vi "stateChange.vi"(8 "error in (no error)":errorcluster, 11 "StaticOutputEditor in":refnum<class "StaticOutputEditor.lvclass">) -> (0 "error out":errorcluster, 3 "StaticOutputEditor out":refnum<class "StaticOutputEditor.lvclass">)   [LabVIEW 2011, in "Views.lvlib" / "ScriptEditor.lvlib" / "StaticOutputEditor.lvclass"]
uses:
  StaticOutputEditor.lvclass
  StaticOutputEditor.lvclass/StaticOutputEditor.ctl
  Tools/DatabaseHelpers/Database Objects/ChannelArray/ChannelArray.lvclass
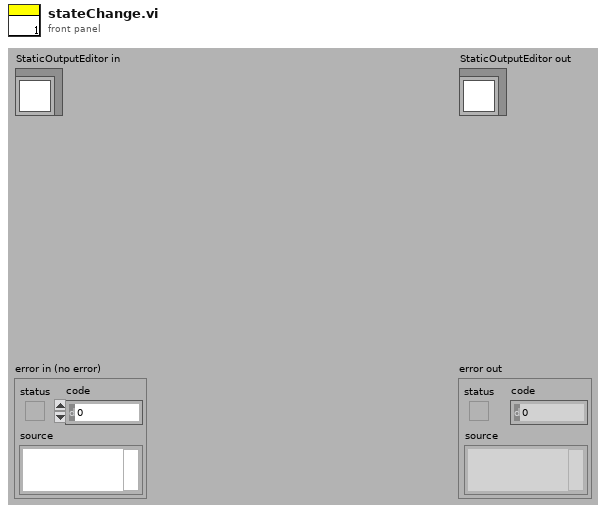
[diagram p1: front panel]
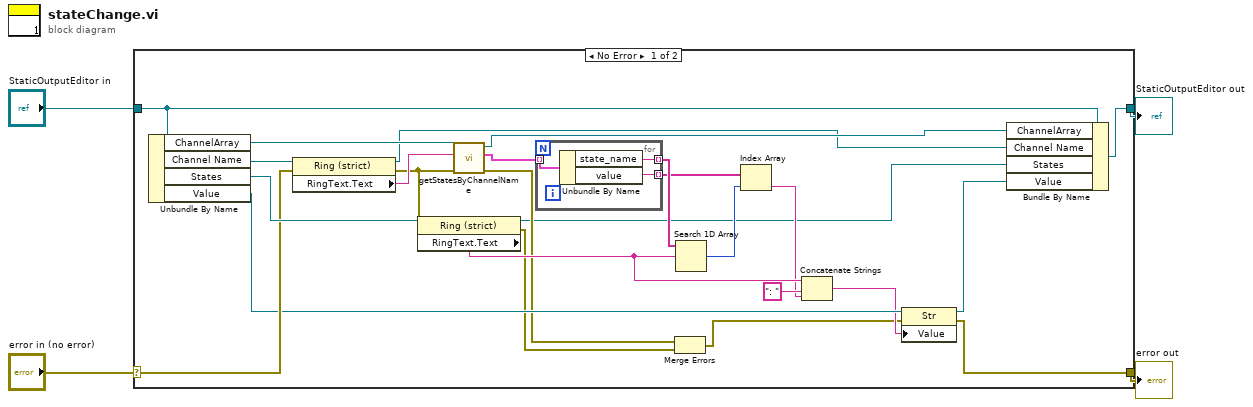
[diagram p0: block diagram]
diagram:
  n1 = case shown="No Error" "error in (no error)" {
    selector: "error in (no error)" -> [w24 w34]
    tunnel: [w11 w34] -> w3
    tunnel: [w5 w33] -> w1
    tunnel: "StaticOutputEditor in" -> [w6 w33]
    frame No Error {
      n2 = Unbundle By Name(w6) -> ("ChannelArray"=w28:refnum<class "ChannelArray.lvclass">, "Channel Name"=w27:refnum<vi>, "States"=w29:refnum<vi>, "Value"=w16:refnum<vi>)
      n3 = property class="Ring (strict)"(reference=w27, error in=w24) -> (reference out=w9:refnum<vi>, error out=w25:errorcluster, "RingText.Text"=w26:string)
      n4 = property class="Ring (strict)"(reference=w29, error in=w25) -> (reference out=w8:refnum<vi>, error out=w13:errorcluster, "RingText.Text"=w19:string)
      n5 = call "getStatesByChannelName.vi"("error in (no error)"=w25, "channel_name"=w26, "ChannelArray in"=w28) -> ("error out"=w14:errorcluster, "states"=w23:cluster{"state_name":string, "value":string}[], "ChannelArray out"=w10:refnum<class "ChannelArray.lvclass">)  [unwired: 6 in]
      n6 = for {
        tunnel: w23 -> [w32] mode=indexing
        tunnel: [w31] -> w22 mode=indexing
        tunnel: [w30] -> w21 mode=indexing
        n7 = Unbundle By Name(w32) -> ("state_name"=w31:string, "value"=w30:string)
      }
      n8 = Merge Errors(w14, w13) -> (w12:errorcluster)
      n9 = Search 1D Array(1D array=w22, element=w19) -> (index of element=w20:i32)  [unwired: 1 in]
      n10 = Index Array(array=w21, index=w20) -> (element=w17:string)
      n11 = Concatenate Strings(w19, ": ", w17) -> (w15:string)
      n12 = property class="Str"(reference=w16, error in=w12, "Value"=w15) -> (reference out=w7:refnum<vi>, error out=w11:errorcluster)
      n13 = Bundle By Name(cluster=w6, "ChannelArray"=w10, "Channel Name"=w9, "States"=w8, "Value"=w7) -> (w5:refnum<class "StaticOutputEditor.lvclass">)
    }
    frame Error {
    }
  }
  "error out" <- w3
  "StaticOutputEditor out" <- w1
